vi "Z6_Beamline.set BB State in GUI.vi"(0 "i ref in":refnum<vi>, 1 "Boolean GUI Ref":refnum<vi>, 2 "Pic GUI Ref":refnum<vi>, 3 "State Status":T1 items=["no info", "off/false/out", "on/true/in", "Failure", "Alarm", "Status 1", "Status 2", "Status 3"], 4 "no Link?":bool, 5 "error in":errorcluster) -> (14 "i ref out":refnum<vi>, 19 "error out":errorcluster)   [LabVIEW 2014, in "Z6_Beamline.lvlib"]
doc: "This VI sets the BB GUI object."
uses:
  Z6_Beamline.lvlib
  PH_StatusHandler/PH_StatusHandler.Status.ctl
  PH_BL-Master/PH_BL-Master.Shutter State.ctl
  PH_Common/Picture/PH_Picture.Alignment.ctl
  PH_Common/PH_Common.lvlib
  PH_Beamline_Common/PH_Beamline_Common.lvlib
  PH_BL-Master/PH_BL-Master.lvlib
  PH_StatusHandler/PH_StatusHandler.lvlib
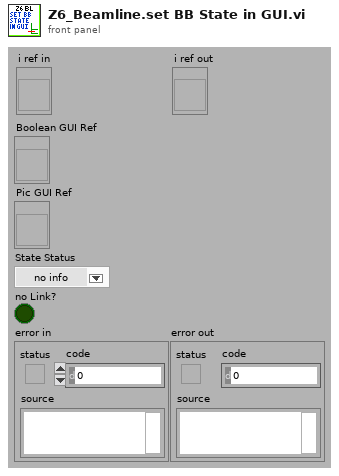
[diagram p1: front panel]
types:
  T1 = typedef "PH_StatusHandler.lvlib/PH_StatusHandler.Status.ctl" = i16
  T2 = typedef "PH_BL-Master.lvlib/PH_BL-Master.Shutter State.ctl" = enum16{"No Link", "No Info", "In", "Out", "in between"}
  T3 = enum16{"No Link", "No Info", "In", "Out", "in between"}
  T4 = typedef "PH_Common.lvlib/PH_Picture.Alignment.ctl" = enum16{"neutral", "left", "right", "up", "down", "vertical", "horizontal", "left down to right up", "left up to right down"}
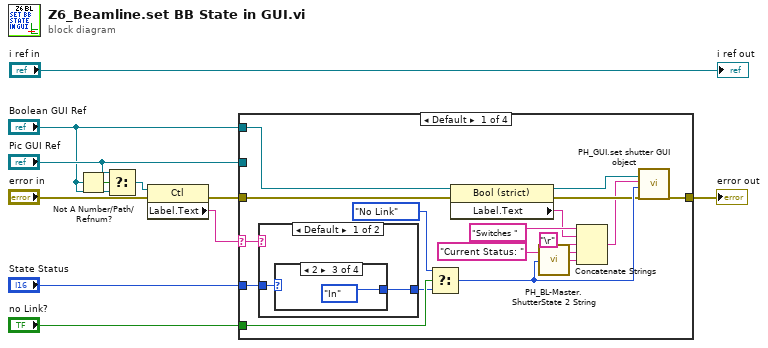
[diagram p0: block diagram]
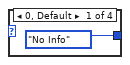
[diagram p2: hidden frame]
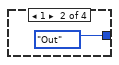
[diagram p3: hidden frame]
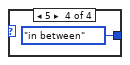
[diagram p4: hidden frame]
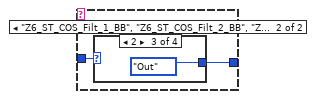
[diagram p5: hidden frame]
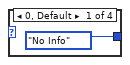
[diagram p6: hidden frame]
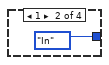
[diagram p7: hidden frame]
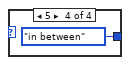
[diagram p8: hidden frame]
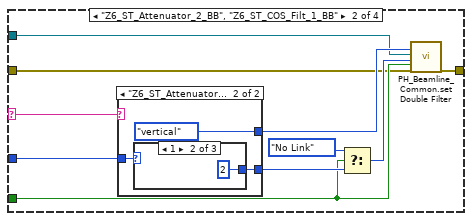
[diagram p9: hidden frame]
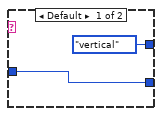
[diagram p10: hidden frame]
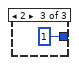
[diagram p12: hidden frame]
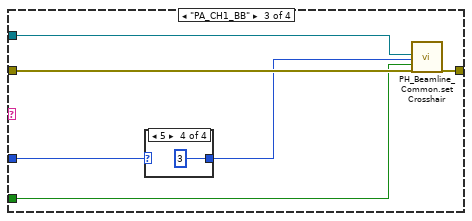
[diagram p13: hidden frame]
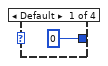
[diagram p14: hidden frame]
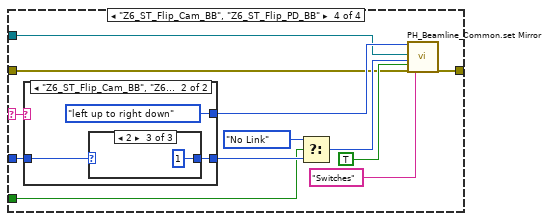
[diagram p17: hidden frame]
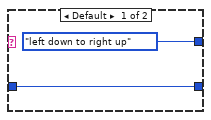
[diagram p18: hidden frame]
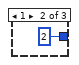
[diagram p20: hidden frame]
diagram:
  n1 = Not A Number/Path/Refnum?(number/path/refnum="Boolean GUI Ref") -> (NaN/Path/Refnum?=w5:bool)
  n2 = Select(t="Pic GUI Ref", s=w5, f="Boolean GUI Ref") -> (s? t:f=w6:refnum<vi>)
  n3 = property class="Ctl"(reference=w6, error in="error in") -> (error out=w7:errorcluster, "Label.Text"=w1:string)  [unwired: 1 out]
  n4 = case shown="Default" w1 {
    selector: w1 -> [w23 w43 _ w71]
    tunnel: [w28 w50 w63 w80] -> w11
    tunnel: w7 -> [w12 w42 w64 w70]
    tunnel: "no Link?" -> [w26 w45 w61 w75]
    tunnel: "State Status" -> [w25 w47 w60 w77]
    tunnel: "Boolean GUI Ref" -> [w21 _ _ _]
    tunnel: "Pic GUI Ref" -> [_ w41 w62 w69]
    frame Default {
      n5 = case shown="Default" w23 {
        tunnel: [w30 w36] -> w24
        tunnel: w25 -> [w29 w35]
        frame Default {
          n6 = case shown="2" w29 {
            tunnel: [PH_BL-Master.Shutter_State."No Info" ("Shutter State") PH_BL-Master.Shutter_State."Out" ("Shutter State") PH_BL-Master.Shutter_State."In" ("Shutter State") PH_BL-Master.Shutter_State."in between" ("Shutter State")] -> w30
            frame 0, Default {
            }
            frame 1 {
            }
            frame 2 {
            }
            frame 5 {
            }
          }
        }
        frame "Z6_ST_COS_Filt_1_BB", "Z6_ST_COS_Filt_2_BB", "Z6_ST_COS_Sensitivity_Switch_BB" {
          n7 = case shown="2" w35 {
            tunnel: [PH_BL-Master.Shutter_State."No Info" ("Shutter State") PH_BL-Master.Shutter_State."In" ("Shutter State") PH_BL-Master.Shutter_State."Out" ("Shutter State") PH_BL-Master.Shutter_State."in between" ("Shutter State")] -> w36
            frame 0, Default {
            }
            frame 1 {
            }
            frame 2 {
            }
            frame 5 {
            }
          }
        }
      }
      n8 = Select(t=PH_BL-Master.Shutter_State."No Link" ("Shutter State"), s=w26, f=w24) -> (s? t:f=w22:T2)
      n9 = property class="Bool (strict)"(reference=w21, error in=w12) -> (reference out=w17:refnum<vi>, error out=w16:errorcluster, "Label.Text"=w14:string)
      n10 = call "PH_BL-Master.ShutterState 2 String.vi"("Shutter State"=w22) -> ("String"=w20:string)
      n11 = Concatenate Strings("Switches " ("string"), w14, "\r", "Current Status: " ("string"), w20) -> (w15:string)
      n12 = call "PH_GUI.set shutter GUI object.vi"("Wanted Boolean Ref"=w17, "Tip Strip"=w15, "Shutter State"=w22, "error in (no error)"=w16) -> ("error out"=w28:errorcluster)  [unwired: 15 in]
    }
    frame "Z6_ST_Attenuator_2_BB", "Z6_ST_COS_Filt_1_BB" {
      n13 = case shown="\"Z6_ST_Attenuator_2_BB\", \"Z6_ST_COS_Filt_2_BB\"" w43 {
        tunnel: [w52 w55] -> w46
        tunnel: w47 -> [w52 w54]
        tunnel: [PH_Picture.Alignment."vertical" ("Alignment (vertical)") PH_Picture.Alignment."vertical" ("Alignment (vertical)")] -> w44
        frame Default {
        }
        frame "Z6_ST_Attenuator_2_BB", "Z6_ST_COS_Filt_2_BB" {
          n14 = case shown="1" w54 {
            selector: w54 -> [w56 _ _]
            tunnel: [w56 u16 2 ("Shutter State") u16 1 ("Shutter State")] -> w55
            frame Default {
            }
            frame 1 {
            }
            frame 2 {
            }
          }
        }
      }
      n15 = Select(t=T3."No Link" ("Shutter State"), s=w45, f=w46) -> (s? t:f=w49:u16)
      n16 = call "PH_Beamline_Common.set Double Filter.vi"("Alignment (vertical)"=w44, "CtlRef"=w41, "State"=w49, "no link"=w45, "error in (no error)"=w42) -> ("error out"=w50:errorcluster)  [unwired: 14 in]
    }
    frame "PA_CH1_BB" {
      n17 = case shown="5" w60 {
        selector: w60 -> [_ w66 w67 _]
        tunnel: [i16 0 ("Cross Hair Status") w66 w67 i16 3 ("Cross Hair Status")] -> w59
        frame Default {
        }
        frame 1 {
        }
        frame 2 {
        }
        frame 5 {
        }
      }
      n18 = call "PH_Beamline_Common.set Crosshair.vi"("CtlRef"=w62, "State"=w59, "no link"=w61, "error in (no error)"=w64) -> ("error out"=w63:errorcluster)  [unwired: 15 in]
    }
    frame "Z6_ST_Flip_Cam_BB", "Z6_ST_Flip_PD_BB" {
      n19 = case shown="\"Z6_ST_Flip_Cam_BB\", \"Z6_ST_Flip_PD_BB\"" w71 {
        tunnel: [w82 w85] -> w76
        tunnel: w77 -> [w82 w84]
        tunnel: [PH_Picture.Alignment."left down to right up" ("Alignment (left down to right up)") PH_Picture.Alignment."left up to right down" ("Alignment (left down to right up)")] -> w73
        frame Default {
        }
        frame "Z6_ST_Flip_Cam_BB", "Z6_ST_Flip_PD_BB" {
          n20 = case shown="2" w84 {
            selector: w84 -> [w86 _ _]
            tunnel: [w86 u16 2 ("Shutter State") u16 1 ("Shutter State")] -> w85
            frame Default {
            }
            frame 1 {
            }
            frame 2 {
            }
          }
        }
      }
      n21 = Select(t=T3."No Link" ("Shutter State"), s=w75, f=w76) -> (s? t:f=w79:u16)
      n22 = call "PH_Beamline_Common.set Mirror.vi"("Alignment (left down to right up)"=w73, "CtlRef"=w69, "Status (on/true/in)"=w79, "GUI Instance does not exist or here?"=TRUE, "error in (no error)"=w70, "Tip Strip (N/A)"="Switches") -> ("error out"=w80:errorcluster)  [unwired: 13 in]
    }
  }
  "error out" <- w11
  "i ref out" <- "i ref in"
